vi "CallProbeVI.vi"(9 "Data":variant, 10 "Probe Name":string, 11 "Probe VI Name":string) -> ()   [LabVIEW 2010]
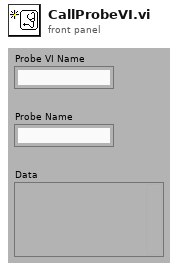
[diagram p1: front panel]
types:
  T1 = enum32{"Invalid", "Standard", "Closed", "Hidden", "Minimized", "Maximized"}
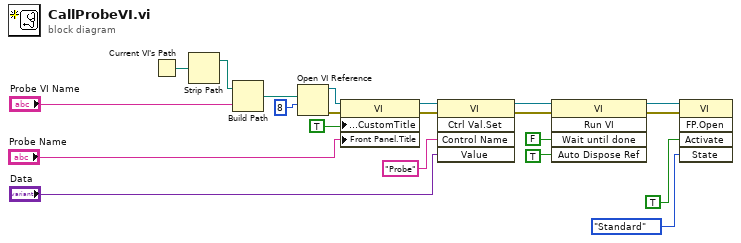
[diagram p0: block diagram]
diagram:
  n1 = Current VI's Path() -> (path=w12:path)
  n2 = Strip Path(path=w12) -> (stripped path=w13:path)  [unwired: 1 out]
  n3 = Build Path(base path=w13, name or relative path="Probe VI Name") -> (appended path=w14:path)
  n4 = Open VI Reference(vi path=w14, options=8) -> (vi reference=w16:refnum<vi>, error out=w19:errorcluster)  [unwired: 4 in]
  n5 = property class="VI"(reference=w16, error in=w19, "Front Panel.CustomTitle"=TRUE ("Front Panel Window:Custom Title"), "Front Panel.Title"="Probe Name") -> (reference out=w17:refnum<vi>, error out=w20:errorcluster)
  n6 = invoke class="VI" method="Ctrl Val.Set"(reference=w17, error in=w20, "Control Name"="Probe" ("control name"), "Value"="Data") -> (reference out=w3:refnum<vi>, error out=w4:errorcluster)  [unwired: 1 in, 3 out]
  n7 = invoke class="VI" method="Run VI"(reference=w3, error in=w4, "Wait until done"=FALSE, "Auto Dispose Ref"=TRUE ("Auto Dispose Reference")) -> (reference out=w6:refnum<vi>, error out=w5:errorcluster)  [unwired: 1 in, 3 out]
  n8 = invoke class="VI" method="FP.Open"(reference=w6, error in=w5, "Activate"=TRUE ("激活？"), "State"=T1."Standard" ("状态")) -> ()  [unwired: 1 in, 5 out]
